vi "Analyze.vi"(8 "error in (no error)":errorcluster, 10 "Image in":T1, 11 "Analyze Energy in":refnum<class "Analyze Energy.lvclass">) -> (0 "error out":errorcluster, 1 "Result":refnum<class "Analyze Results Base.lvclass">, 2 "Image out":T1, 3 "Analyze Energy out":refnum<class "Analyze Energy.lvclass">)   [LabVIEW 2020, in "Analyze.lvlib" / "Analyze Energy.lvclass"]
uses:
  Analyze Energy.lvclass
  C:/POLARIS Programme/POLARIS-AS-3-Cams/Submodules/HIJ Vision/Analyze/Analyze Classes/Analyze BaseClass/Analyze BaseClass/Analyze BaseClass.lvclass
  <vilib>/vision/Image Controls.llb/IMAQ Image.ctl
  Results and Overlays/Results Base/Analyze Results Base.lvclass
  Results and Overlays/Results Total Counts/Analyze Results Total Counts.lvclass
  Analyze Parameter/Analyze Parameter Energy per Count/Analyze Parameter Energy per Count.lvclass
  C:/POLARIS Programme/POLARIS-AS-3-Cams/Submodules/HIJ Vision/Analyze/Analyze Parameter/Analyze Parameter Base/Analyze Parameter Base.lvclass
  Results and Overlays/Results Energy/Analyze Results Energy.lvclass
  C:/POLARIS Programme/POLARIS-AS-3-Cams/Submodules/HIJ Vision/Analyze/Results and Overlays/Results Base/Analyze Results Base.lvclass
  C:/POLARIS Programme/POLARIS-AS-3-Cams/Submodules/HIJ Vision/Analyze/Results and Overlays/Results Total Counts/Analyze Results Total Counts.lvclass
  Results and Overlays/Results Total Counts/Analyze Results Total Counts.lvclass/Analyze Results Total Counts.ctl
  Analyze Parameter/Analyze Parameter Energy per Count/Analyze Parameter Energy per Count.lvclass/Analyze Parameter Energy per Count.ctl
  Results and Overlays/Results Energy/Analyze Results Energy.lvclass/Analyze Results Energy.ctl
  Results and Overlays/Results Total Counts/Read Total Counts.vi
  Analyze Parameter/Analyze Parameter Energy per Count/Read J_count.vi
  Results and Overlays/Results Energy/Write Energy.vi
  Results and Overlays/Results Total Counts/Write Total Counts.vi
  Analyze Total Counts/Analyze Total Counts.lvclass
  Analyze BaseClass/Analyze BaseClass/Analyze BaseClass.lvclass
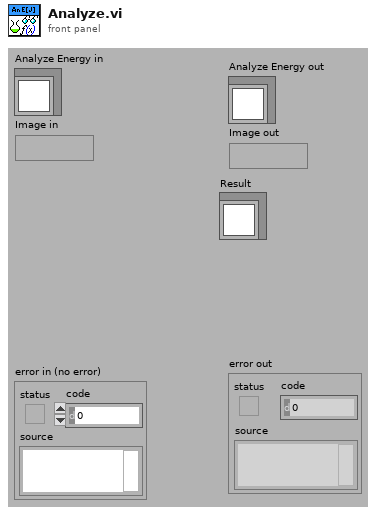
[diagram p1: front panel]
types:
  T1 = typedef "IMAQ Image.ctl" = refnum<image>
  T2 = typedef "ROI Descriptor" = cluster{"Global Rectangle":i32[], "Contours":cluster{"ID":enum32{"External", "Internal"}, "Type":u32, "Coordinates":i32[]}[]}
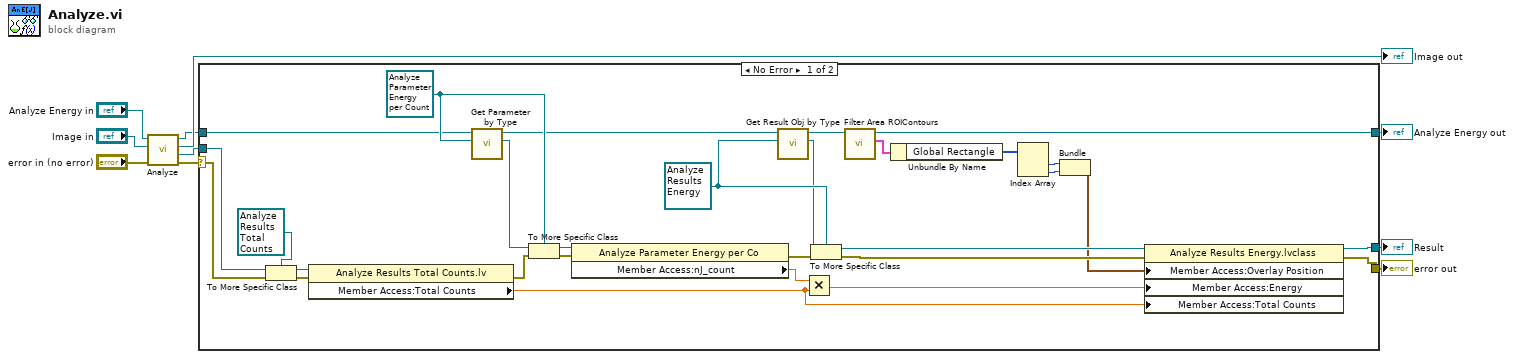
[diagram p0: block diagram]
diagram:
  n1 = call-parent "Analyze.vi"("error in (no error)"="error in (no error)", "Image in"="Image in", "Analyze Total Counts in"="Analyze Energy in") -> ("error out"=w1:errorcluster, "Result"=w5:refnum<class "Analyze Results Base.lvclass">, "Image out"=→"Image out":T1, "Analyze Total Counts out"=w9:refnum<class "Analyze Energy.lvclass">)  [unwired: 5 in]
  n2 = case shown="No Error" w1 {
    selector: w1 -> [w24 w40]
    tunnel: w9 -> [w37 w42]
    tunnel: w5 -> [w35 w41]
    tunnel: [w18 w42] -> w4
    tunnel: [w32 w41] -> w3
    tunnel: [w31 w40] -> w2
    frame No Error {
      w39 = refnum<class "Analyze Results Energy.lvclass"> refnum ("Analyze Results Energy.lvclass")
      w38 = refnum<class "Analyze Parameter Energy per Count.lvclass"> refnum ("Analyze Parameter Energy per Count.lvclass")
      n3 = To More Specific Class(target class=refnum<class "Analyze Results Total Counts.lvclass"> refnum ("Analyze Results Total Counts.lvclass"), reference=w35, error in=w24) -> (specific class reference=w30:refnum<class "Analyze Results Total Counts.lvclass">, error out=w27:errorcluster)
      n4 = property class="Analyze Results Total Counts.lv"(reference=w30, error in=w27) -> (error out=w26:errorcluster, "Member Access:Total Counts"=w13:dbl)  [unwired: 1 out]
      n5 = call "Get Parameter by Type.vi"("Parameter Type"=w38, "Analyze BaseClass in"=w37) -> ("Parameter"=w33:refnum<class "Analyze Parameter Base.lvclass">, "Analyze BaseClass out"=w34:refnum<class "Analyze Energy.lvclass">)  [unwired: 6 in, 2 out]
      n6 = To More Specific Class(target class=w38, reference=w33, error in=w26) -> (specific class reference=w29:refnum<class "Analyze Parameter Energy per Count.lvclass">, error out=w25:errorcluster)
      n7 = property class="Analyze Parameter Energy per Co"(reference=w29, error in=w25) -> (error out=w21:errorcluster, "Member Access:nJ_count"=w28:dbl[unit])  [unwired: 1 out]
      n8 = call "Get Result Obj by Type.vi"("Parameter Type"=w39, "Analyze BaseClass in"=w34) -> ("Parameter"=w22:refnum<class "Analyze Results Base.lvclass">, "Analyze BaseClass out"=w19:refnum<class "Analyze Energy.lvclass">)  [unwired: 6 in, 2 out]
      n9 = Multiply(x=w28, y=w13) -> (x*y=w11:dbl[unit])
      n10 = To More Specific Class(target class=w39, reference=w22, error in=w21) -> (specific class reference=w23:refnum<class "Analyze Results Energy.lvclass">, error out=w20:errorcluster)
      n11 = call-dynamic "Filter Area ROIContours.vi"("Analyze BaseClass in"=w19) -> ("ROI of Area type"=w17:T2, "Analyze BaseClass out"=w18:refnum<class "Analyze Energy.lvclass">)  [unwired: 8 in, 1 out]
      n12 = Unbundle By Name(w17) -> ("Global Rectangle"=w16:i32[])
      n13 = Index Array(array=w16) -> (element #1=w14:i32, element #2=w15:i32)  [unwired: 2 in]
      n14 = Bundle(w14, w15) -> (w12:cluster{i32, i32})  [unwired: 1 in]
      n15 = property class="Analyze Results Energy.lvclass"(reference=w23, error in=w20, "Member Access:Overlay Position"=w12, "Member Access:Energy"=w11, "Member Access:Total Counts"=w13) -> (reference out=w32:refnum<class "Analyze Results Energy.lvclass">, error out=w31:errorcluster)
    }
    frame Error {
    }
  }
  "error out" <- w2
  "Analyze Energy out" <- w4
  "Result" <- w3
